vi "Image Processing Handler Module.vi"() -> ()   [LabVIEW 2018]
panel:
  out "Image":T1(plugin-control)
  in  "Video File":path
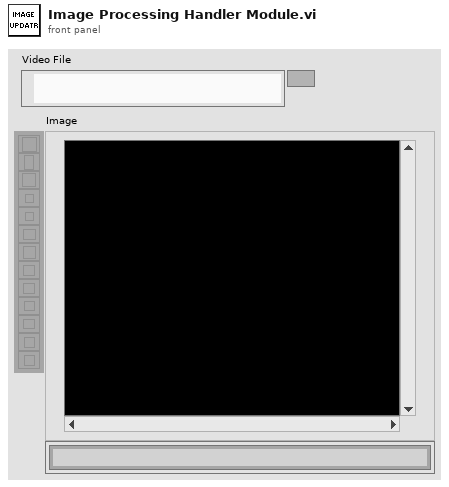
[diagram p1: front panel]
types:
  T1 = typedef "IMAQ Image.ctl" = refnum<image>
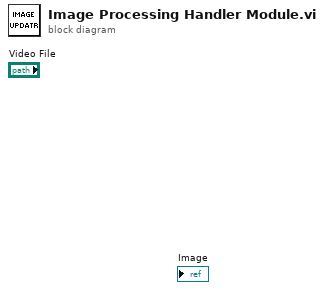
[diagram p0: block diagram]
diagram:
